vi "PS1-_GND_Connection.vi"(0 "On/Off":bool, 1 "Delay Time (s)":dbl=1.0, 3 "error in":errorcluster) -> (10 "error out":errorcluster)   [LabVIEW 2015]
panel:
  # "ON means close relay\nOFF means open relay"
  # "port1/line7"
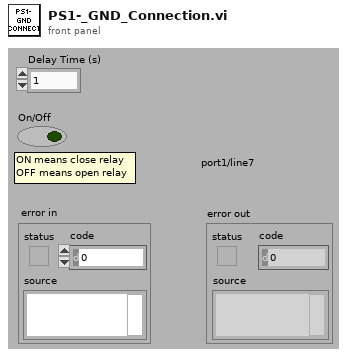
[diagram p1: front panel]
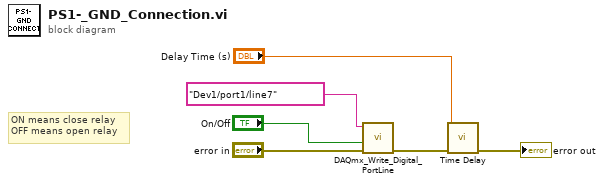
[diagram p0: block diagram]
diagram:
  # "ON means close relay\nOFF means open relay"
  n1 = call "DAQmx_Write_Digital_PortLine.vi"("Device/Ports/Lines"="Dev1/port1/line7", "Boolean"="On/Off", "error in"="error in") -> ("error out"=w4:errorcluster)  [unwired: 6 in, 1 out]
  n2 = call "Time Delay"("error in (no error)"=w4, "Delay Time (s)"="Delay Time (s)") -> ("error out"=→"error out":errorcluster)  [unwired: 9 in]
